vi "Max Search.vi"() -> ()   [LabVIEW 2021]
panel:
  in  "Number of Iterations":dbl
  out "Random Number":dbl
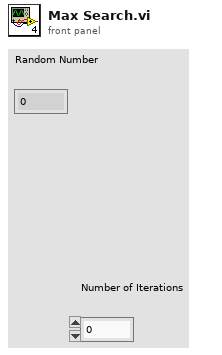
[diagram p1: front panel]
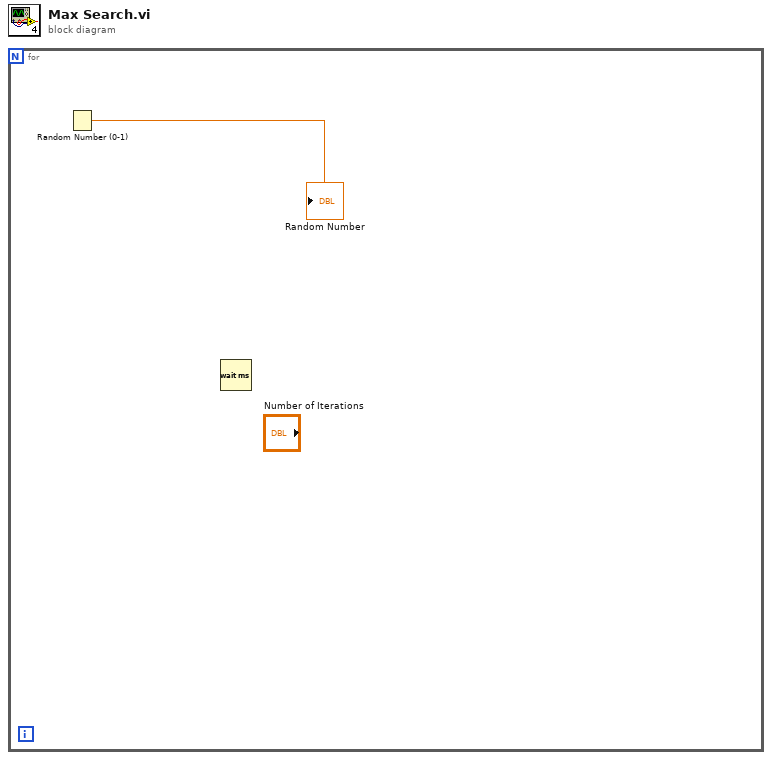
[diagram p0: block diagram]
diagram:
  n1 = for {
    n2 = Random Number (0-1)() -> (number: 0 to 1=→"Random Number":dbl)
    n3 = Wait (ms)() -> ()  [unwired: 1 in, 1 out]
  }
